vi "G_Estados_Elevador.vi"() -> ()   [LabVIEW 2020]
panel:
  out "Estados_Elevador":cluster{"Masa elevador":bool, "Elevador":bool}={"Masa elevador"=TRUE, "Elevador"=FALSE}
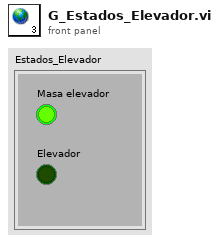
[diagram p1: front panel]
diagram:
